vi "Invert DIR.vi"(10 "direction in":bool, 11 "Invert DIR?":bool) -> (3 "direction out":bool)   [LabVIEW 2014]
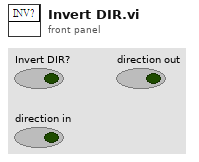
[diagram p1: front panel]
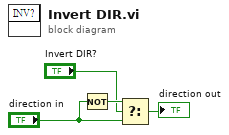
[diagram p0: block diagram]
diagram:
  n1 = Not(x="direction in") -> (.not. x?=w4:bool)
  n2 = Select(t=w4, s="Invert DIR?", f="direction in") -> (s? t:f=→"direction out":bool)
